vi "ping.vi"(8 "error in (no error)":errorcluster, 11 "address":string[](array[string])=["192.168.10.20"]) -> (0 "error out":errorcluster, 2 "standard output":string, 3 "ping":bool)   [LabVIEW 2017]
uses:
  <vilib>/regexp/Match Regular Expression.xnode
panel:
  out "concatenated string":string
  out "offset past match 2":i32
  out "return code":i32
  out "standard error":string
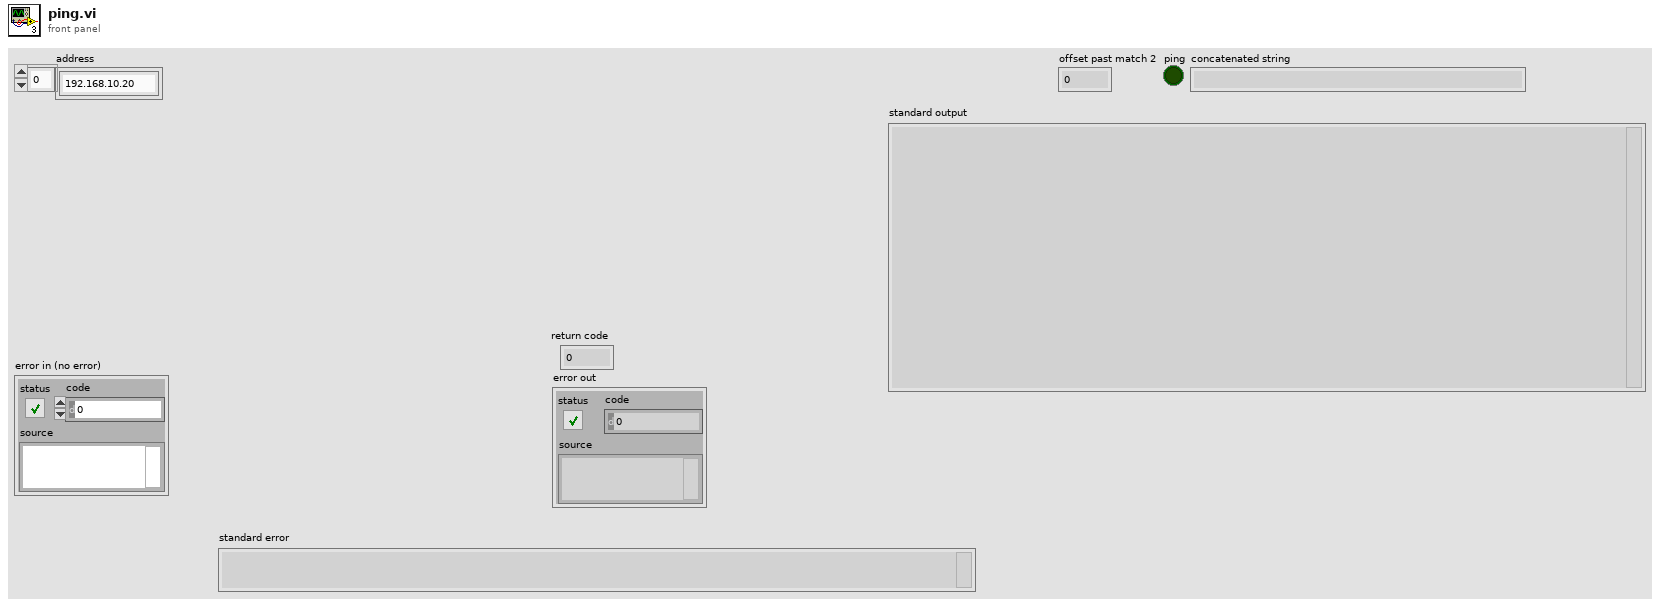
[diagram p1: front panel]
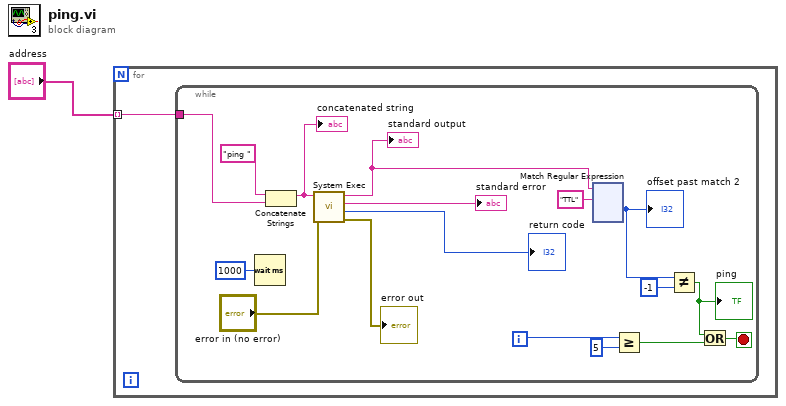
[diagram p0: block diagram]
diagram:
  n1 = for {
    tunnel: "address" -> [w2] mode=indexing
    n2 = while {
      tunnel: w2 -> [w16]
      i -> [w7]
      stop <- w8 stop-if-true
      n3 = Wait (ms)(milliseconds to wait=u32 1000) -> ()  [unwired: 1 out]
      n4 = Concatenate Strings("ping " ("string"), w16) -> (w17:string)
      "concatenated string" <- w17
      n5 = call <vilib>:"System Exec.vi"("error in (no error)"="error in (no error)", "command line"=w17) -> ("error out"=→"error out":errorcluster, "return code"=→"return code":i32, "standard error"=→"standard error":string, "standard output"=w3:string)  [unwired: 6 in]
      "standard output" <- w3
      n6 = xnode "Match Regular Expression"("input string"=w3, "regular expression"="TTL") -> ("offset past match"=w12:i32)  [unwired: 4 in, 4 out]
      "offset past match 2" <- w12
      n7 = Greater Or Equal?(x=w7, y=5) -> (x >= y?=w6:bool)
      n8 = Not Equal?(x=w12, y=-1) -> (x != y?=w9:bool)
      "ping" <- w9
      n9 = Or(x=w9, y=w6) -> (x .or. y?=w8:bool)
    }
  }
